vi "string_to_mV.vi"(11 "Received HEX":string) -> (1 "LSB byte":u8, 2 "MSB byte":u8, 3 "Voltage mV":dbl)   [LabVIEW 2012]
panel:
  out "Voltage mV 2":dbl
  out "LSB byte 2":u8
  out "MSB byte 2":u8
  out "<ACK>":u8
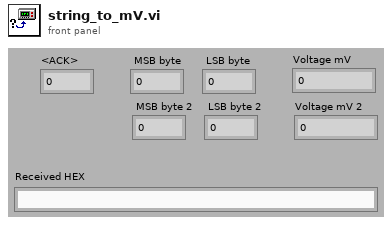
[diagram p1: front panel]
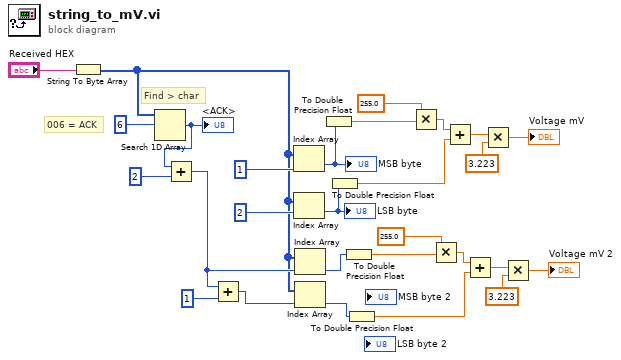
[diagram p0: block diagram]
diagram:
  # "006 = ACK"
  # "Find > char"
  n1 = String To Byte Array(string="Received HEX") -> (unsigned byte array=w10:u8[])
  n2 = Search 1D Array(1D array=w10, element=6) -> (index of element=w15:i32)  [unwired: 1 out]
  "<ACK>" <- w15
  n3 = Add(x=w15, y=2) -> (x+y=w13:i32)
  n4 = Add(x=w13, y=1) -> (x+y=w11:i32)
  n5 = Index Array(array=w10, index=1) -> (element=w27:u8)
  "MSB byte" <- w27
  n6 = Index Array(array=w10, index=2) -> (element=w26:u8)
  "LSB byte" <- w26
  n7 = Index Array(array=w10, index=w13) -> (element=w2:u8)
  n8 = Index Array(array=w10, index=w11) -> (element=w1:u8)
  n9 = To Double Precision Float(number=w27) -> (double precision float=w24:dbl)
  n10 = To Double Precision Float(number=w26) -> (double precision float=w22:dbl)
  n11 = To Double Precision Float(number=w2) -> (double precision float=w8:dbl)
  n12 = To Double Precision Float(number=w1) -> (double precision float=w6:dbl)
  n13 = Multiply(x=255.0, y=w24) -> (x*y=w23:dbl)
  n14 = Multiply(x=255.0, y=w8) -> (x*y=w7:dbl)
  n15 = Add(x=w23, y=w22) -> (x+y=w20:dbl)
  n16 = Add(x=w7, y=w6) -> (x+y=w4:dbl)
  n17 = Multiply(x=w20, y=3.223) -> (x*y=→"Voltage mV":dbl)
  n18 = Multiply(x=w4, y=3.223) -> (x*y=→"Voltage mV 2":dbl)
